vi "Configure Output Sweep.vi"(0 "VISA resource name":refnum<visa-resource-name>, 1 "Source Mode  (0: Voltage)":u16(ring) items=["Voltage", "Current"], 2 "Sweep Direction  (0: Ascending)":u16(ring) items=["Ascending", "Descending"], 5 "Number of Points (5)":u32=5, 7 "Minimum Amplitude (1)":dbl=1.0, 9 "Maximum Amplitude (2)":dbl=2.0, 11 "error in (no error)":errorcluster, 12 "Sweep Spacing  (0: Linear)":u16(ring) items=["Linear", "Logarithmic"]) -> (4 "VISA resource name out":refnum<visa-resource-name>, 15 "error out":errorcluster)   [LabVIEW 2019, in "Keithley 24XX.lvlib"]
doc: "Configures the range, direction, and unit scale of an upcoming output sweep."
uses:
  Keithley 24XX.lvlib
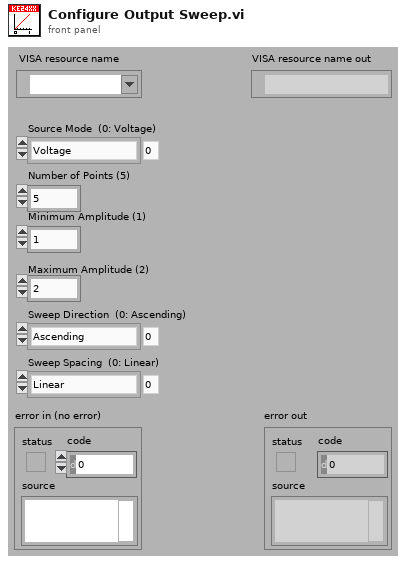
[diagram p1: front panel]
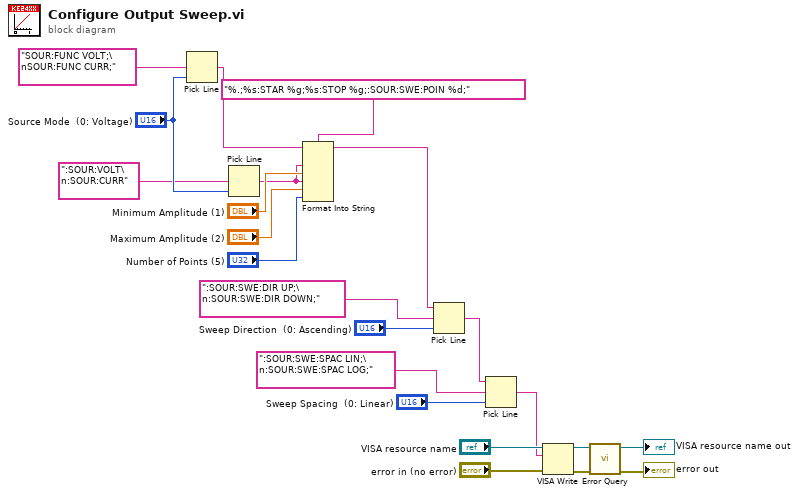
[diagram p0: block diagram]
diagram:
  n1 = Pick Line(multi-line string="SOUR:FUNC VOLT;\nSOUR:FUNC CURR;", line index="Source Mode  (0: Voltage)") -> (output string=w15:string)  [unwired: 1 in]
  n2 = Pick Line(multi-line string=":SOUR:VOLT\n:SOUR:CURR" ("string (\"\")"), line index="Source Mode  (0: Voltage)") -> (output string=w17:string)  [unwired: 1 in]
  n3 = Format Into String(format string="%.;%s:STAR %g;%s:STOP %g;:SOUR:SWE:POIN %d;", initial string=w15, w17, "Minimum Amplitude (1)", w17, "Maximum Amplitude (2)", "Number of Points (5)") -> (resulting string=w9:string)  [unwired: 1 in, 1 out]
  n4 = Pick Line(string ("")=w9, multi-line string=":SOUR:SWE:DIR UP;\n:SOUR:SWE:DIR DOWN;", line index="Sweep Direction  (0: Ascending)") -> (output string=w8:string)
  n5 = Pick Line(string ("")=w8, multi-line string=":SOUR:SWE:SPAC LIN;\n:SOUR:SWE:SPAC LOG;", line index="Sweep Spacing  (0: Linear)") -> (output string=w5:string)
  n6 = VISA Write(VISA resource name="VISA resource name", write buffer=w5, error in (no error)="error in (no error)") -> (VISA resource name out=w4:refnum<visa-resource-name>, error out=w3:errorcluster)  [unwired: 1 out]
  n7 = call "Error Query.vi"("error in (no error)"=w3, "VISA resource name"=w4) -> ("error out"=→"error out":errorcluster, "VISA resource name out"=→"VISA resource name out":refnum<visa-resource-name>)  [unwired: 6 in, 2 out]
